vi "Switch Heater Status No Check (Read).vi"(6 "ISOBUS address":T2=-1 caption="ISOBUS address (-1)", 8 "error in":errorcluster, 11 "Mercury Reference In":T3) -> (0 "error out":errorcluster, 2 "Switch Heater Status":string, 3 "Mercury Reference Out":T3, 4 "Valid?":T1)   [LabVIEW 2013, in "Mercury iXX.lvlib" / "Magnet.lvlib"]
doc: "Acquire the most recent switch heater status."
uses:
  <instrlib>/Mercury iXX/Public/Libraries/Magnet.lvlib
  <instrlib>/Mercury iXX/Public/Controls/Mercury Reference.ctl
  <instrlib>/Mercury iXX/Public/Controls/Comms Transport Layer.ctl
  <instrlib>/Mercury iXX/Private/Controls/Query Dynamic Reference.ctl
  <instrlib>/Mercury iXX/Public/Controls/ISOBus Address.ctl
  <instrlib>/Mercury iXX/Public/Controls/Is Valid LED.ctl
  <instrlib>/Mercury iXX/Private/Controls/Command Verbs.ctl
  <instrlib>/Mercury iXX/Mercury iXX.lvlib
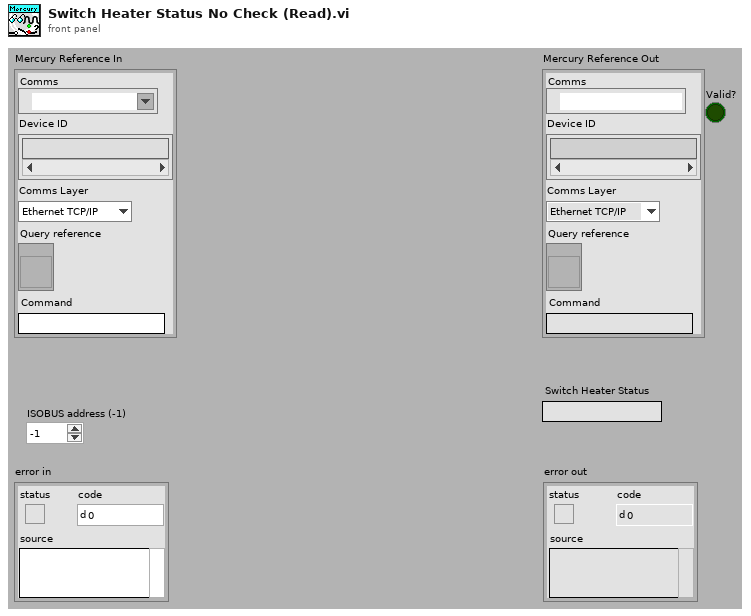
[diagram p1: front panel]
types:
  T1 = typedef "Mercury iXX.lvlib/Is Valid LED.ctl" = bool
  T2 = typedef "Mercury iXX.lvlib/ISOBus Address.ctl" = i32
  T3 = typedef "Mercury iXX.lvlib/Mercury Reference.ctl" = cluster{"Comms":refnum<visa-resource-name>, "Device ID":string[], "Comms Layer":T4, "Command":string, "Query reference":T5}
  T4 = typedef "Mercury iXX.lvlib/Comms Transport Layer.ctl" = enum16{"Ethernet TCP/IP", "USB", "ISOBus - RS-232", "GPIB"}
  T5 = typedef "Mercury iXX.lvlib/Query Dynamic Reference.ctl" = refnum<vi>
  T6 = typedef "Mercury iXX.lvlib/Command Verbs.ctl" = string
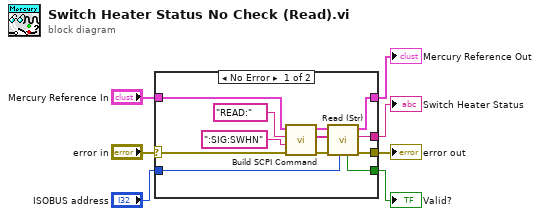
[diagram p0: block diagram]
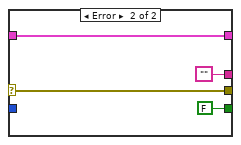
[diagram p2: hidden frame]
diagram:
  n1 = case shown="No Error" "error in" {
    selector: "error in" -> [w8 w23]
    tunnel: "ISOBUS address" -> [w19 _]
    tunnel: [w18 T1 FALSE ("Valid?")] -> w6
    tunnel: [w17 w23] -> w5
    tunnel: [w16 w22] -> w4
    tunnel: [w15 ""] -> w3
    tunnel: "Mercury Reference In" -> [w12 w22]
    frame No Error {
      n2 = call <instrlib>:"Build SCPI Command.vi"("error in"=w8, "Noun(s)"=":SIG:SWHN" ("Command"), "Verb"=T6 "READ:", "Mercury Reference In"=w12) -> ("error out"=w10:errorcluster, "SCPI Message(s)"=w9:string[], "Mercury Reference Out"=w11:T3)  [unwired: 5 out]
      n3 = call <instrlib>:"Read (Str).vi"("ISOBUS address"=w19, "error in"=w10, "SCPI Message(s)"=w9, "Mercury Reference In"=w11) -> ("error out"=w17:errorcluster, "Response"=w15:string, "Mercury Reference Out"=w16:T3, "Valid?"=w18:T1)  [unwired: 4 out]
    }
    frame Error {
    }
  }
  "Mercury Reference Out" <- w4
  "error out" <- w5
  "Valid?" <- w6
  "Switch Heater Status" <- w3
